vi "BuildRtTarget.vi"(8 "error in (no error)":errorcluster, 11 "Library Builder in":refnum<class "Library Builder.lvclass">) -> (0 "error out":errorcluster, 3 "Library Builder out":refnum<class "Library Builder.lvclass">)   [LabVIEW 2020, in "Library Builder.lvclass"]
uses:
  Library Builder.lvclass
  Library Builder.lvclass/Library Builder.ctl
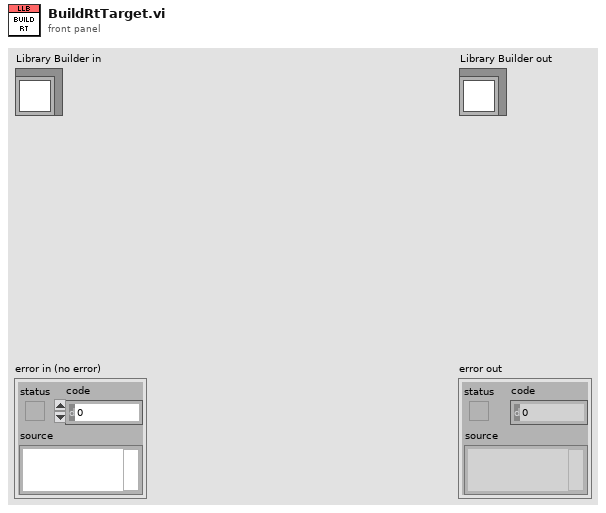
[diagram p1: front panel]
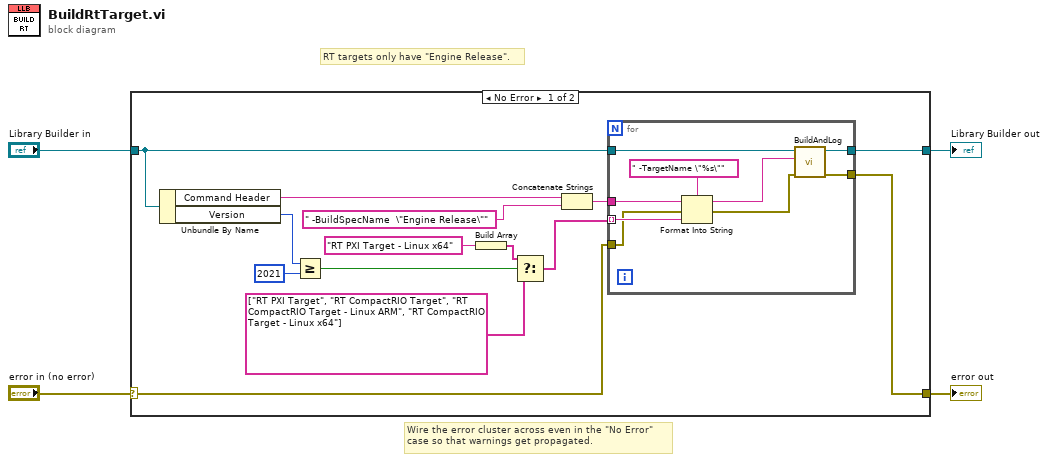
[diagram p0: block diagram]
diagram:
  # "Wire the error cluster across even in the \"No Error\"\ncase so that warnings get propagated."
  # "RT targets only have \"Engine Release\"."
  n1 = case shown="No Error" "error in (no error)" {
    selector: "error in (no error)" -> [w12 w29]
    tunnel: [w17 w29] -> w3
    tunnel: [w18 w28] -> w1
    tunnel: "Library Builder in" -> [w16 w28]
    frame No Error {
      n2 = Unbundle By Name(w16) -> ("Command Header"=w15:string, "Version"=w10:u32)
      n3 = Greater Or Equal?(x=w10, y=u32 2021 ("Version")) -> (x >= y?=w8:bool)
      n4 = Build Array("RT PXI Target - Linux x64") -> (w7:string[])
      n5 = Select(t=w7, s=w8, f=string[] ["RT PXI Target", "RT CompactRIO Target", "RT CompactRIO Target - Linux ARM", "RT CompactRIO Target - Linux x64"]) -> (s? t:f=w5:string[])
      n6 = Concatenate Strings(w15, " -BuildSpecName  \"Engine Release\"") -> (w13:string)
      n7 = for {
        tunnel: [w26] -> w17
        tunnel: w16 -> [w25]
        tunnel: [w27] -> w18
        tunnel: w13 -> [w24]
        tunnel: w5 -> [w23] mode=indexing
        tunnel: w12 -> [w22]
        n8 = Format Into String(format string=" -TargetName \"%s\"", initial string=w24, error in=w22, w23) -> (resulting string=w21:string, error out=w20:errorcluster)
        n9 = call "BuildAndLog.vi"("error in (no error)"=w20, "Command In"=w21, "Library Builder in"=w25) -> ("error out"=w26:errorcluster, "Library Builder out"=w27:refnum<class "Library Builder.lvclass">)  [unwired: 7 in]
      }
    }
    frame Error {
    }
  }
  "error out" <- w3
  "Library Builder out" <- w1
